vi "Build DashBoard Data.vi"(11 "Dashboard Enables":T3={"Analog Module 1"=[TRUE, TRUE, TRUE, TRUE, TRUE, TRUE, TRUE, TRUE], "Analog Module 2"=[FALSE, FALSE, FALSE, FALSE, FALSE, FALSE, FALSE, FALSE], "Digital Module 1"=TRUE, "Digital Module 2"=FALSE, "Solenoid Module"=TRUE}) -> ()   [LabVIEW 2011]
doc: "This VI builds data and sends it back to the dashboard PC program. By default it sends back the raw values for the first analog, digital, and solenoid module. Modify it to send back the data you want to view. Consider adding higher level data to the Dashboard Datatype.ctl and to this VI. Then update the Dashboard to display the data however you like.\n\nThis software is licensed. Open the labview\\readme\\WPI Robotics Library Open Source License.txt file for more information."
uses:
  DashboardEnable.ctl
  Dashboard Datatype.ctl
  <vilib>/Rock Robotics/WPI/DriverStation/WPI_DriverStationDigitalData.ctl
  <vilib>/Rock Robotics/WPI/DriverStation/DriverStationLCD/WPI_DriverStationLCDLCDLine.ctl
  Actual RPM Global.vi
  Robot Global Data.vi
panel:
  out "Dashboard Data":T1
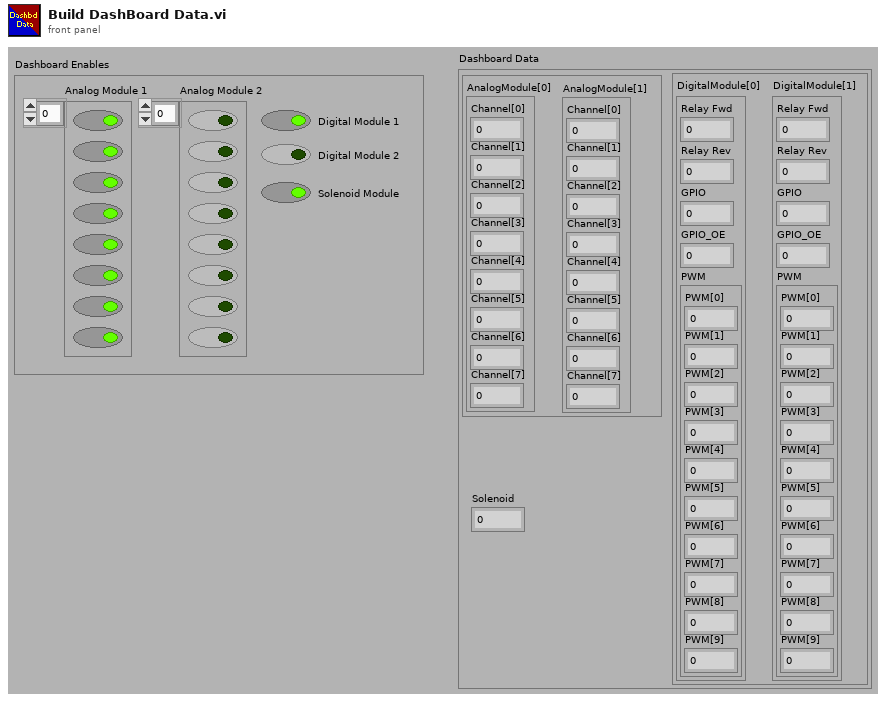
[diagram p1: front panel]
types:
  T1 = typedef "Dashboard Datatype.ctl" = cluster{cluster{"AnalogModule[0]":cluster{"Channel[0]":sgl, "Channel[1]":sgl, "Channel[2]":sgl, "Channel[3]":sgl, "Channel[4]":sgl, "Channel[5]":sgl, "Channel[6]":sgl, "Channel[7]":sgl}, "AnalogModule[1]":cluster{"Channel[0]":sgl, "Channel[1]":sgl, "Channel[2]":sgl, "Channel[3]":sgl, "Channel[4]":sgl, "Channel[5]":sgl, "Channel[6]":sgl, "Channel[7]":sgl}}, cluster{"DigitalModule[0]":T2, "DigitalModule[1]":T2}, "Solenoid":u8}
  T2 = typedef "WPI_DriverStationDigitalData.ctl" = cluster{"Relay Fwd":u8, "Relay Rev":u8, "GPIO":u16, "GPIO_OE":u16, "PWM":cluster{"PWM[0]":u8, "PWM[1]":u8, "PWM[2]":u8, "PWM[3]":u8, "PWM[4]":u8, "PWM[5]":u8, "PWM[6]":u8, "PWM[7]":u8, "PWM[8]":u8, "PWM[9]":u8}}
  T3 = typedef "DashboardEnable.ctl" = cluster{"Analog Module 1":bool[], "Analog Module 2":bool[], "Digital Module 1":bool, "Digital Module 2":bool, "Solenoid Module":bool}
  T4 = typedef "WPI_DriverStationLCDLCDLine.ctl" = enum16{"Main - Line 1", "User - Line 2", "User - Line 3", "User - Line 4", "User - Line 5", "User - Line 6"}
  T5 = cluster{"Position":cluster{"X":dbl, "Y":dbl}, "Distance (ft)":dbl}[]
  T6 = cluster{"Target Info[0]":cluster{"Position":cluster{"X":dbl, "Y":dbl}, "Distance (ft)":dbl}, "Target Info[1]":cluster{"Position":cluster{"X":dbl, "Y":dbl}, "Distance (ft)":dbl}, "Target Info[2]":cluster{"Position":cluster{"X":dbl, "Y":dbl}, "Distance (ft)":dbl}, "Target Info[3]":cluster{"Position":cluster{"X":dbl, "Y":dbl}, "Distance (ft)":dbl}, "Target Info[4]":cluster{"Position":cluster{"X":dbl, "Y":dbl}, "Distance (ft)":dbl}, "Target Info[5]":cluster{"Position":cluster{"X":dbl, "Y":dbl}, "Distance (ft)":dbl}, "Target Info[6]":cluster{"Position":cluster{"X":dbl, "Y":dbl}, "Distance (ft)":dbl}, "Target Info[7]":cluster{"Position":cluster{"X":dbl, "Y":dbl}, "Distance (ft)":dbl}, "Target Info[8]":cluster{"Position":cluster{"X":dbl, "Y":dbl}, "Distance (ft)":dbl}}
  T7 = cluster{"AnalogModule[0]":cluster{"Channel[0]":sgl, "Channel[1]":sgl, "Channel[2]":sgl, "Channel[3]":sgl, "Channel[4]":sgl, "Channel[5]":sgl, "Channel[6]":sgl, "Channel[7]":sgl}, "AnalogModule[1]":cluster{"Channel[0]":sgl, "Channel[1]":sgl, "Channel[2]":sgl, "Channel[3]":sgl, "Channel[4]":sgl, "Channel[5]":sgl, "Channel[6]":sgl, "Channel[7]":sgl}}
  T8 = cluster{"Channel[0]":sgl, "Channel[1]":sgl, "Channel[2]":sgl, "Channel[3]":sgl, "Channel[4]":sgl, "Channel[5]":sgl, "Channel[6]":sgl, "Channel[7]":sgl}[]
  T9 = cluster{"Channel[0]":sgl, "Channel[1]":sgl, "Channel[2]":sgl, "Channel[3]":sgl, "Channel[4]":sgl, "Channel[5]":sgl, "Channel[6]":sgl, "Channel[7]":sgl}
  T10 = cluster{"AnalogModule[0][0]":sgl, "AnalogModule[0][1]":sgl, "AnalogModule[0][2]":sgl, "AnalogModule[0][3]":sgl, "AnalogModule[0][4]":sgl, "AnalogModule[0][5]":sgl, "AnalogModule[0][6]":sgl, "AnalogModule[0][7]":sgl}
  T11 = cluster{"[0]":cluster{"Channel[0]":sgl, "Channel[1]":sgl, "Channel[2]":sgl, "Channel[3]":sgl, "Channel[4]":sgl, "Channel[5]":sgl, "Channel[6]":sgl, "Channel[7]":sgl}, "[1]":cluster{"Channel[0]":sgl, "Channel[1]":sgl, "Channel[2]":sgl, "Channel[3]":sgl, "Channel[4]":sgl, "Channel[5]":sgl, "Channel[6]":sgl, "Channel[7]":sgl}}
  T12 = cluster{"DigitalModule[0]":T2, "DigitalModule[1]":T2}
  T13 = typedef "FPGA_DIODevRef.ctl" = cluster{"DevStatus":errorcluster, "Module":T14}
  T14 = typedef "FPGA_TypedefDigitalModule.ctl" = enum16{"Digital Module 1", "Digital Module 2"}
  T15 = cluster{"[0]":u8, "[1]":u8, "[2]":u8, "[3]":u8, "[4]":u8, "[5]":u8, "[6]":u8, "[7]":u8, "[8]":u8, "[9]":u8}
  T16 = typedef "FPGA_SolenoidDevRef.ctl" = cluster{"DevStatus":errorcluster, "Module":T17}
  T17 = typedef "FPGA_TypedefSolenoidModule.ctl" = enum16{"Solenoid Module 1", "Solenoid Module 2"}
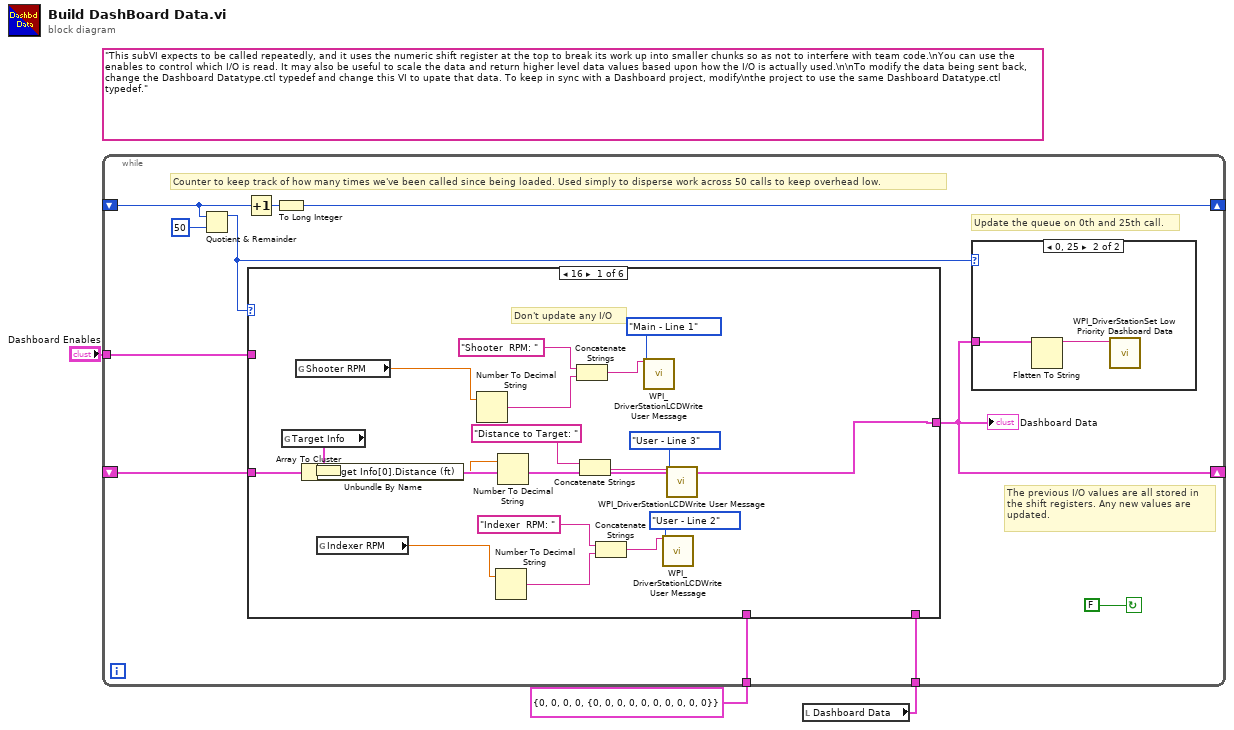
[diagram p0: block diagram]
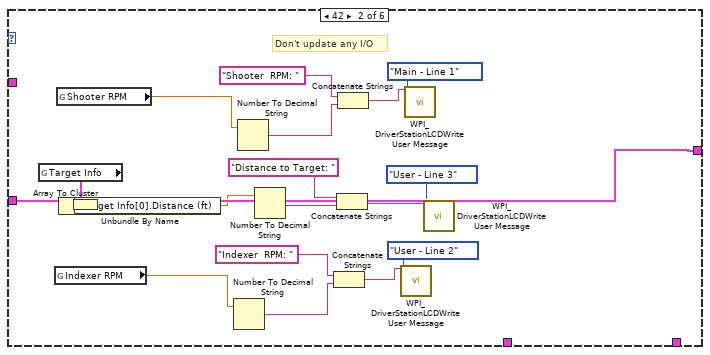
[diagram p3: hidden frame]
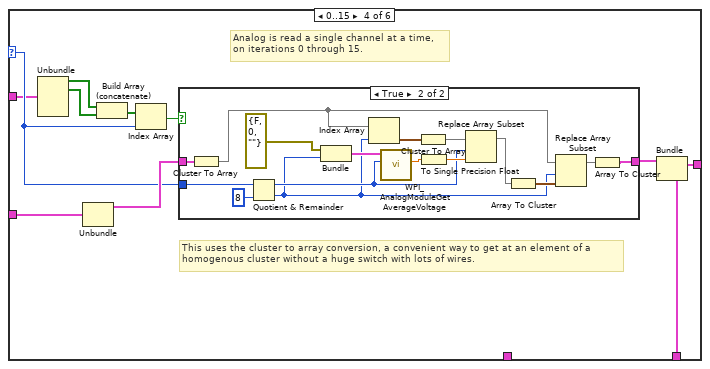
[diagram p5: hidden frame]
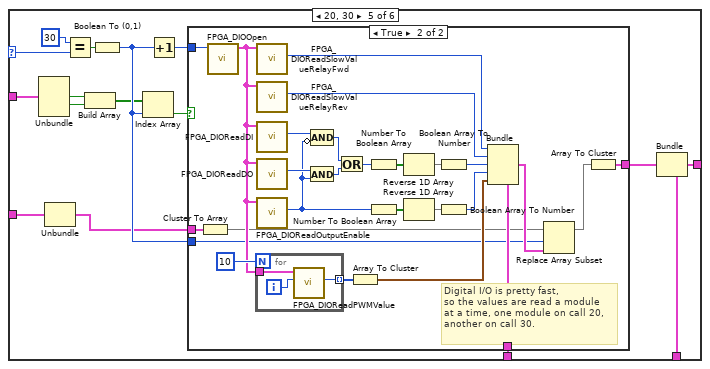
[diagram p7: hidden frame]
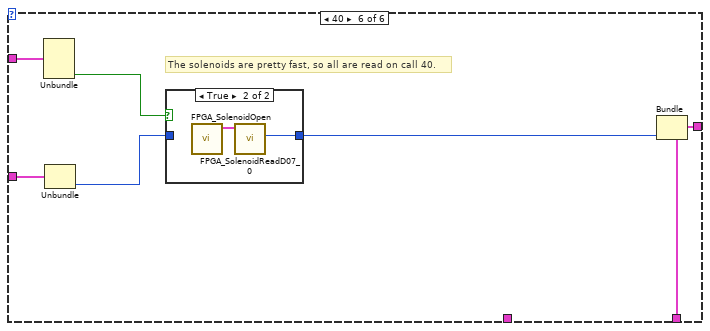
[diagram p9: hidden frame]
diagram:
  (unwired) "This subVI expects to be called repeatedly, and it uses the numeric shift register at the top to break its work up into smaller chunks so as not to interfere with team code.\nYou can use the enables to control which I/O is read. It may also be useful to scale the data and return higher level data values based upon how the I/O is actually used.\n\nTo modify the data being sent back, change the Dashboard Datatype.ctl typedef and change this VI to upate that data. To keep in sync with a Dashboard project, modify\nthe project to use the same Dashboard Datatype.ctl typedef."
  n1 = local read "Dashboard Data"() -> (w2:T1)
  n2 = while {
    shift-right: [w7] -> _
    shift-left: _ -> [w9]
    shift-right: [w4] -> _
    shift-left: _ -> [w12]
    tunnel: T2 {"Relay Fwd"=0, "Relay Rev"=0, "GPIO"=0, "GPIO_OE"=0, "PWM"={"PWM[0]"=0, "PWM[1]"=0, "PWM[2]"=0, "PWM[3]"=0, "PWM[4]"=0, "PWM[5]"=0, "PWM[6]"=0, "PWM[7]"=0, "PWM[8]"=0, "PWM[9]"=0}} ("DigitalModule[1]") -> [w11]
    tunnel: w2 -> [w6]
    tunnel: "Dashboard Enables" -> [w5]
    stop <- FALSE continue-if-true
    # "Counter to keep track of how many times we've been called since being loaded. Used simply to disperse work across 50 calls to keep overhead low."
    # "Update the queue on 0th and 25th call."
    # "The previous I/O values are all stored in\nthe shift registers. Any new values are\nupdated."
    n3 = Quotient & Remainder(x=w9, y=50) -> (x-y*floor(x/y)=w8:i32)  [unwired: 1 out]
    n4 = Increment(x=w9) -> (x+1=w14:i32)
    n5 = case shown="16" w8 {
      selector: w8 -> [_ _ _ w59 w91 _]
      tunnel: [w34 w52 w53 w55 w82 w131] -> w4
      tunnel: w12 -> [w34 w52 w53 w54 w84 w133]
      tunnel: w11 -> [_ _ _ _ w97 _]
      tunnel: w6 -> [_ _ _ w61 w83 w130]
      tunnel: w5 -> [_ _ _ w58 w89 w134]
      frame 16 {
        # "Don't update any I/O"
        n6 = global read "Robot Global Data.vi" "Target Info"() -> (w28:T5)
        n7 = global read "Actual RPM Global.vi" "Shooter RPM"() -> (w30:dbl)
        n8 = Array To Cluster(array=w28) -> (cluster=w27:T6)
        n9 = Unbundle By Name(w27) -> ("Target Info[0].Distance (ft)"=w26:dbl)
        n10 = global read "Actual RPM Global.vi" "Indexer RPM"() -> (w18:dbl)
        n11 = Number To Decimal String(number=w30) -> (decimal integer string=w29:string)  [unwired: 1 in]
        n12 = Number To Decimal String(number=w18) -> (decimal integer string=w17:string)  [unwired: 1 in]
        n13 = Number To Decimal String(number=w26) -> (decimal integer string=w25:string)  [unwired: 1 in]
        n14 = Concatenate Strings("Shooter  RPM: ", w29) -> (w32:string)
        n15 = Concatenate Strings("Distance to Target: " ("string"), w25) -> (w22:string)
        n16 = Concatenate Strings("Indexer  RPM: ", w17) -> (w20:string)
        n17 = call <vilib>:"WPI_DriverStationLCDWrite User Message.vi"("line text"=w32, "line"=WPI_DriverStationLCDLCDLine."Main - Line 1") -> ()  [unwired: 13 in, 1 out]
        n18 = call <vilib>:"WPI_DriverStationLCDWrite User Message.vi"("line text"=w20, "line"=WPI_DriverStationLCDLCDLine."User - Line 2") -> ()  [unwired: 13 in, 1 out]
        n19 = call <vilib>:"WPI_DriverStationLCDWrite User Message.vi"("line text"=w22, "line"=WPI_DriverStationLCDLCDLine."User - Line 3") -> ()  [unwired: 13 in, 1 out]
      }
      frame 42 {
        # "Don't update any I/O"
        n20 = global read "Robot Global Data.vi" "Target Info"() -> (w46:T5)
        n21 = global read "Actual RPM Global.vi" "Indexer RPM"() -> (w36:dbl)
        n22 = global read "Actual RPM Global.vi" "Shooter RPM"() -> (w48:dbl)
        n23 = Array To Cluster(array=w46) -> (cluster=w45:T6)
        n24 = Unbundle By Name(w45) -> ("Target Info[0].Distance (ft)"=w44:dbl)
        n25 = Number To Decimal String(number=w36) -> (decimal integer string=w35:string)  [unwired: 1 in]
        n26 = Number To Decimal String(number=w48) -> (decimal integer string=w47:string)  [unwired: 1 in]
        n27 = Number To Decimal String(number=w44) -> (decimal integer string=w43:string)  [unwired: 1 in]
        n28 = Concatenate Strings("Indexer  RPM: ", w35) -> (w38:string)
        n29 = Concatenate Strings("Distance to Target: " ("string"), w43) -> (w40:string)
        n30 = Concatenate Strings("Shooter  RPM: ", w47) -> (w50:string)
        n31 = call <vilib>:"WPI_DriverStationLCDWrite User Message.vi"("line text"=w38, "line"=WPI_DriverStationLCDLCDLine."User - Line 2") -> ()  [unwired: 13 in, 1 out]
        n32 = call <vilib>:"WPI_DriverStationLCDWrite User Message.vi"("line text"=w50, "line"=WPI_DriverStationLCDLCDLine."Main - Line 1") -> ()  [unwired: 13 in, 1 out]
        n33 = call <vilib>:"WPI_DriverStationLCDWrite User Message.vi"("line text"=w40, "line"=WPI_DriverStationLCDLCDLine."User - Line 3") -> ()  [unwired: 13 in, 1 out]
      }
      frame Default {
      }
      frame 0..15 {
        # "This uses the cluster to array conversion, a convenient way to get at an element of a\nhomogenous cluster without a huge switch with lots of wires."
        # "Analog is read a single channel at a time,\non iterations 0 through 15."
        n34 = Unbundle(w58) -> ("Analog Module 1"=w57:bool[], "Analog Module 2"=w56:bool[])  [unwired: 3 out]
        n35 = Unbundle(w54) -> (w60:T7)  [unwired: 2 out]
        n36 = Build Array (concatenate)(w57, w56) -> (w63:bool[])
        n37 = Index Array(array=w63, index=w59) -> (element=w64:bool)
        n38 = case shown="True" w64 {
          tunnel: w59 -> [_ w72]
          tunnel: [w65 w69] -> w62
          tunnel: w60 -> [w65 w68]
          frame False {
          }
          frame True {
            n39 = Cluster To Array(cluster=w68) -> (array=w67:T8)
            n40 = Quotient & Remainder(x=w72, y=8) -> (x-y*floor(x/y)=w71:i32, floor(x/y)=w66:i32)
            n41 = Bundle("DevStatus"=errorcluster {"status"=FALSE, "code"=0, "source"=""}, w66) -> (w80:cluster{"DevStatus":errorcluster, i32})  [unwired: 1 out]
            n42 = Index Array(array=w67, index=w66) -> (element=w74:T9)
            n43 = call <vilib>:"WPI_AnalogModuleGetAverageVoltage.vi"("Channel"=w71, "AnalogModuleDevStatus"=w80) -> ("Average Voltage"=w77:dbl)  [unwired: 1 in, 8 out]
            n44 = Cluster To Array(cluster=w74) -> (array=w73:sgl[])
            n45 = To Single Precision Float(number=w77) -> (single precision float=w76:sgl)
            n46 = Replace Array Subset(array=w73, new element=w76, index=w71) -> (w75:sgl[])
            n47 = Array To Cluster(array=w75) -> (cluster=w79:T10)
            n48 = Replace Array Subset(array=w67, new element=w79, index=w66) -> (w70:T8)
            n49 = Array To Cluster(array=w70) -> (cluster=w69:T11)
          }
        }
        n50 = Bundle(cluster=w61, w62) -> (w55:T1)  [unwired: 2 out]
      }
      frame 20, 30 {
        n51 = Unbundle(w89) -> ("Digital Module 1"=w88:bool, "Digital Module 2"=w87:bool)  [unwired: 3 out]
        n52 = Unbundle(w84) -> (w86:T12)  [unwired: 2 out]
        n53 = Equal?(x=30, y=w91) -> (x = y?=w95:bool)
        n54 = Build Array(w88, w87) -> (w90:bool[])
        n55 = Boolean To (0,1)(Boolean=w95) -> (0, 1=w93:i16)
        n56 = Index Array(array=w90, index=w93) -> (element=w92:bool)
        n57 = Increment(x=w93) -> (x+1=w94:i16)
        n58 = case shown="True" w92 {
          tunnel: w97 -> [_ w106]
          tunnel: [w98 w99] -> w85
          tunnel: w94 -> [_ w104]
          tunnel: w93 -> [_ w103]
          tunnel: w86 -> [w98 w102]
          frame False {
          }
          frame True {
            # "Digital I/O is pretty fast,\nso the values are read a module\nat a time, one module on call 20,\nanother on call 30."
            n59 = Cluster To Array(cluster=w102) -> (array=w101:T2[])
            n60 = call <vilib>:"FPGA_DIOOpen.vi"("Module (Module 1)"=w104) -> ("DIODeviceRef"=w122:T13)  [unwired: 1 in, 9 out]
            n61 = for {
              N: 10 -> [_]
              tunnel: w122 -> [w127]
              tunnel: [w125] -> w123 mode=indexing
              i -> [w126]
              n62 = call <vilib>:"FPGA_DIOReadPWMValue.vi"("PWMChannel"=w126, "DIODeviceRef In"=w127) -> ("PWMValue"=w125:u8)  [unwired: 1 in, 8 out]
            }
            n63 = call <vilib>:"FPGA_DIOReadSlowValueRelayFwd.vi"("DIODeviceRef In"=w122) -> ("Relay Forward"=w115:u8)  [unwired: 1 in, 9 out]
            n64 = call <vilib>:"FPGA_DIOReadSlowValueRelayRev.vi"("DIODeviceRef In"=w122) -> ("Relay Reverse"=w116:u8)  [unwired: 1 in, 9 out]
            n65 = call <vilib>:"FPGA_DIOReadDI.vi"("DIODeviceRef In"=w122) -> ("DI"=w120:u16)  [unwired: 1 in, 9 out]
            n66 = call <vilib>:"FPGA_DIOReadDO.vi"("DIODeviceRef In"=w122) -> ("DO"=w119:u16)  [unwired: 1 in, 9 out]
            n67 = call <vilib>:"FPGA_DIOReadOutputEnable.vi"("DIODeviceRef In"=w122) -> ("OutputEnable"=w110:u16)  [unwired: 1 in, 9 out]
            n68 = And(x=w119, y=w110) -> (x .and. y?=w118:u16)
            n69 = Compound Arithmetic op=AND(w120, invert w110) -> (w117:u16)
            n70 = Or(x=w117, y=w118) -> (x .or. y?=w108:u16)
            n71 = Array To Cluster(array=w123) -> (cluster=w121:T15)
            n72 = Number To Boolean Array(number=w108) -> (Boolean array=w113:bool[])
            n73 = Number To Boolean Array(number=w110) -> (Boolean array=w112:bool[])
            n74 = Reverse 1D Array(array=w113) -> (reversed array=w114:bool[])
            n75 = Reverse 1D Array(array=w112) -> (reversed array=w111:bool[])
            n76 = Boolean Array To Number(Boolean array=w114) -> (number=w107:u32)
            n77 = Boolean Array To Number(Boolean array=w111) -> (number=w109:u32)
            n78 = Bundle(cluster=w106, "Relay Fwd"=w115, "Relay Rev"=w116, "GPIO"=w107, "GPIO_OE"=w109, "PWM"=w121) -> (w105:T2)
            n79 = Replace Array Subset(array=w101, new element=w105, index=w103) -> (w100:T2[])
            n80 = Array To Cluster(array=w100) -> (cluster=w99:cluster{"[0]":T2, "[1]":T2})
          }
        }
        n81 = Bundle(cluster=w83, w85) -> (w82:T1)  [unwired: 2 out]
      }
      frame 40 {
        # "The solenoids are pretty fast, so all are read on call 40."
        n82 = Unbundle(w134) -> ("Solenoid Module"=w128:bool)  [unwired: 4 out]
        n83 = Unbundle(w133) -> ("Solenoid"=w132:u8)  [unwired: 2 out]
        n84 = case shown="True" w128 {
          tunnel: [w135 w136] -> w129
          tunnel: w132 -> [w135 _]
          frame False {
          }
          frame True {
            n85 = call <vilib>:"FPGA_SolenoidOpen.vi"() -> ("SolenoidDevRef"=w137:T16)  [unwired: 2 in, 9 out]
            n86 = call <vilib>:"FPGA_SolenoidReadD07_0.vi"("SolenoidDevRef"=w137) -> ("DO7:0"=w136:u8)  [unwired: 1 in, 9 out]
          }
        }
        n87 = Bundle(cluster=w130, "Solenoid"=w129) -> (w131:T1)  [unwired: 2 out]
      }
    }
    "Dashboard Data" <- w4
    n88 = To Long Integer(number=w14) -> (32bit integer=w7:i32)
    n89 = case shown="0, 25" w8 {
      tunnel: w4 -> [_ w16]
      frame Default {
      }
      frame 0, 25 {
        n90 = Flatten To String(anything=w16) -> (data string=w15:string)  [unwired: 1 in, 4 out]
        n91 = call <vilib>:"WPI_DriverStationSet Low Priority Dashboard Data.vi"("User Data"=w15) -> ()  [unwired: 1 in, 10 out]
      }
    }
  }
